vi "niRFUtil ERR Check Valid Input (wfm).vi"   [LabVIEW 2015, in "niRFUtil.lvlib"]
uses:
  niRFUtil.lvlib
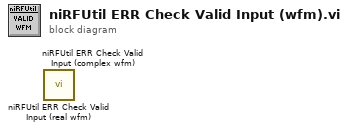
[diagram p0: block diagram]
diagram:
  n1 = call "niRFUtil ERR Check Valid Input (real wfm).vi"() -> ()  [unwired: 10 in, 2 out]
  n2 = call "niRFUtil ERR Check Valid Input (complex wfm).vi"() -> ()  [unwired: 10 in, 2 out]
